vi "Undistort.vi"(0 "image in":refnum<class "MSC Image.lvclass">, 1 "camMatrix":dbl[][](array[numeric]) caption="(fx, 0, cx;\n 0, fy, cy;\n 0, 0, 1)", 2 "distMatrix":dbl[](array[numeric]) caption="(k1, k2, p1, p2, k3)", 5 "error in (no error)":errorcluster) -> (14 "image out":refnum<class "MSC Image.lvclass">, 15 "camMatrix out":dbl[][](array[numeric]) caption="(fx, 0, cx;\n 0, fy, cy;\n 0, 0, 1)", 19 "error out":errorcluster)   [LabVIEW 2014, in "MSC Image.lvclass"]
doc: "After the estimation of the cam matrix and distort matrix is done, it is possible to undistort an image.\n\nFor more information about this process please check the documentation."
uses:
  MSC Image.lvclass
  MSC Image.lvclass/MSC Image.ctl
  Dependencies/x86/MSC I Process32.dll
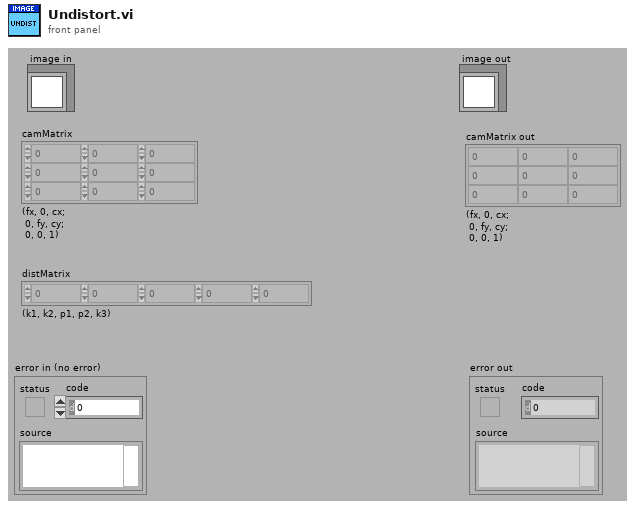
[diagram p1: front panel]
types:
  T1 = typedef "Image.ctl" = cluster{"Pointer":u64, "Size":T2, "Image Type":T3, "Time Stamp":timestamp, "Variant":variant}
  T2 = typedef "Size.ctl" = cluster{"Cols":i32, "Rows":i32}
  T3 = typedef "Image Type.ctl" = i32
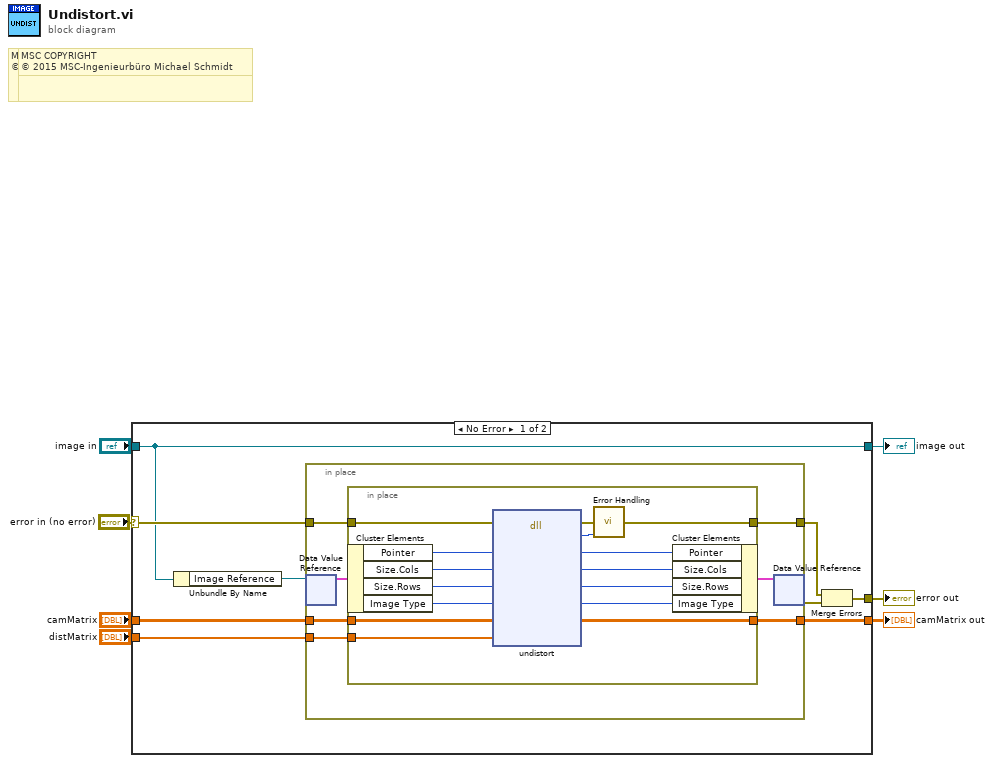
[diagram p0: block diagram]
diagram:
  # "MSC COPYRIGHT\n© 2016 MSC-Ingenieurbüro Michael Schmidt"
  # "MSC COPYRIGHT\n© 2016 MSC-Ingenieurbüro Michael Schmidt"
  # "MSC COPYRIGHT\n© 2015 MSC-Ingenieurbüro Michael Schmidt"
  # "MSC COPYRIGHT\n© 2015 MSC-Ingenieurbüro Michael Schmidt"
  n1 = case shown="No Error" "error in (no error)" {
    selector: "error in (no error)" -> [w10 w40]
    tunnel: [w14 w40] -> w4
    tunnel: [w9 w39] -> w6
    tunnel: "image in" -> [w9 w39]
    tunnel: "distMatrix" -> [w13 _]
    tunnel: "camMatrix" -> [w12 _]
    tunnel: [w11 _] -> w1
    frame No Error {
      n2 = Unbundle By Name(w9) -> ("Image Reference"=w8:refnum<data-value>)
      n3 = in-place {
        in-place-border: w10 -> [w21]
        in-place-border: [w20] -> w15
        in-place-border: w13 -> [w19]
        in-place-border: w12 -> [w18]
        in-place-border: [w17] -> w11
        n4 = in-place-dvr #1(w8) -> (w22:T1)  [unwired: 1 out]
        n5 = in-place {
          in-place-border: w21 -> [w31]
          in-place-border: [w38] -> w20
          in-place-border: w19 -> [w26]
          in-place-border: w18 -> [w25]
          in-place-border: [w24] -> w17
          n6 = in-place-cluster #2(w22) -> ("Pointer"=w37:u64, "Size.Cols"=w36:i32, "Size.Rows"=w35:i32, "Image Type"=w28:T3)
          n7 = dll-call lib="C:/Users/MSC/LabVIEW Projekte/LV 2014/MSC I-Process/user.lib/MSC-I Process/Dependencies/x86/MSC I Process*.dll" fn="undistort"(error in=w31, "pointer"=w37, "cols"=w36, "rows"=w35, "type"=w28, "camMatrix"=w25, "distMatrix"=w26) -> (error out=w30:errorcluster, "error"=w29:i32, "pointer"=w34:u64, "cols"=w33:i32, "rows"=w32:i32, "type"=w27:i32, "camMatrix"=w24:dbl[][])  [unwired: 3 in, 1 out]
          n8 = call "Error Handling.vi"("error in (no error)"=w30, "return type"=w29) -> ("error out"=w38:errorcluster)  [unwired: 12 in, 1 out]
          n9 = in-place-cluster #2("Pointer"=w34, "Size.Cols"=w33, "Size.Rows"=w32, "Image Type"=w27) -> (w23:T1)
        }
        n10 = in-place-dvr #1(w23) -> (w16:errorcluster)  [unwired: 1 out]
      }
      n11 = Merge Errors(w15, w16) -> (w14:errorcluster)
    }
    frame Error {
    }
  }
  "error out" <- w4
  "image out" <- w6
  "camMatrix out" <- w1
